vi "WriteCSV.vi"(6 "波形":dbl[][](array[numeric]), 7 "通用数据":string[](array[string]), 9 "任务编号":string, 10 "时间":string, 11 "file path (dialog if empty)":path caption="文件路径 （空时为对话框）") -> ()   [LabVIEW 2018]
uses:
  <vilib>/Utility/file.llb/Write Delimited Spreadsheet (string).vi
  <vilib>/Utility/file.llb/Write Delimited Spreadsheet (DBL).vi
  <vilib>/Utility/file.llb/Read Delimited Spreadsheet (string).vi
panel:
  out "子数组":string[][](array[string])
  out "all rows":string[][](array[string]) caption="所有行"
  # "写入CSV文件\n判断是否需要重新写入还是继续写入"
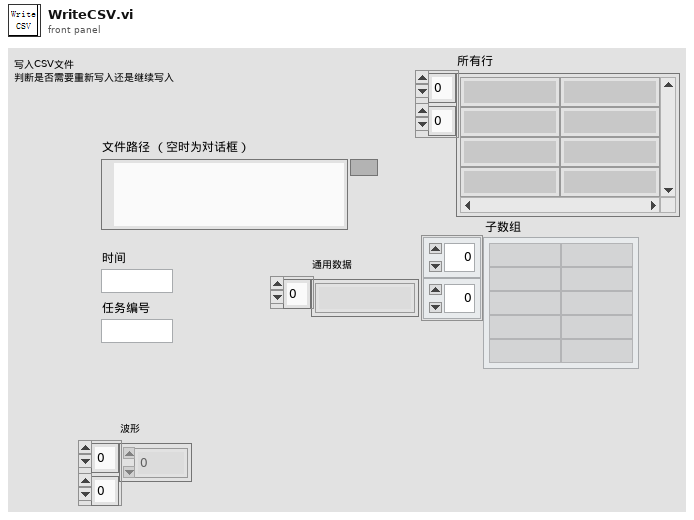
[diagram p1: front panel]
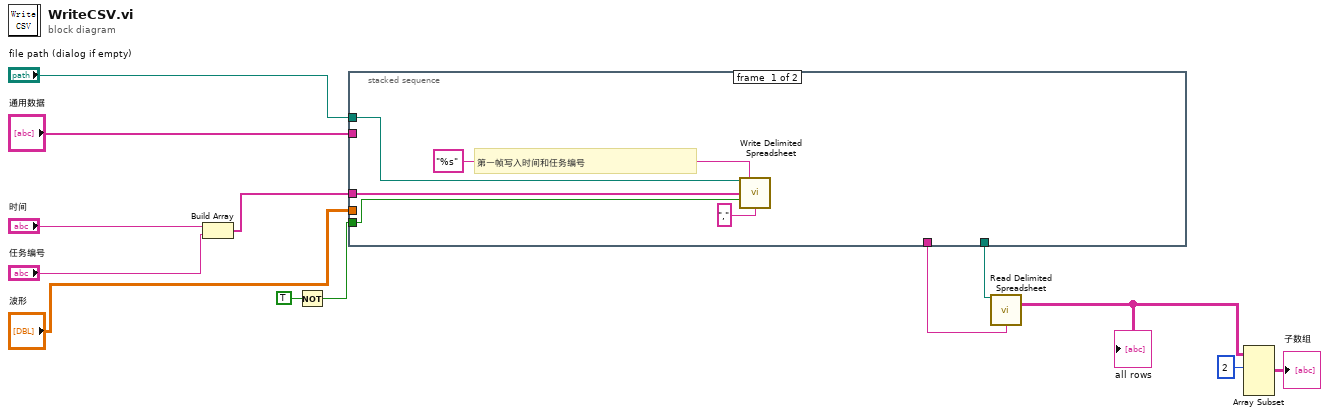
[diagram p0: block diagram]
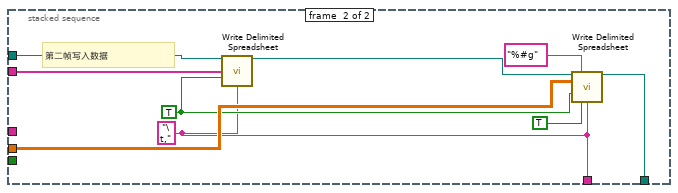
[diagram p2: hidden frame]
diagram:
  n1 = Build Array("时间", "任务编号") -> (w1:string[])
  n2 = Not(x=TRUE ("是否重新写入")) -> (.not. x?=w9:bool)
  n3 = stacked-sequence {
    tunnel: "file path (dialog if empty)" -> [w18 w24]
    tunnel: w9 -> [w16 _]
    tunnel: "波形" -> [_ w27]
    tunnel: "通用数据" -> [_ w25]
    tunnel: [_ w21] -> w6
    tunnel: [_ w19] -> w5
    tunnel: w1 -> [w14 _]
    frame #0 {
      # "第一帧写入时间和任务编号"
      n4 = call-poly <vilib>:"Write Delimited Spreadsheet.vi"("file path (dialog if empty)"=w18, "format (%s)"="%s", "1D data"=w14, "append to file? (new file:F)"=w16, "delimiter (\\t)"="," ("delimiter (\\t)")) -> ()  [unwired: 9 in, 2 out]
    }
    frame #1 {
      w19 = "\t," ("delimiter (\\t)")
      w22 = TRUE ("append to file? (new file:F)")
      # "第二帧写入数据"
      n5 = call-poly <vilib>:"Write Delimited Spreadsheet.vi"("file path (dialog if empty)"=w24, "1D data"=w25, "append to file? (new file:F)"=w22, "delimiter (\\t)"=w19) -> ("new file path (Not A Path if cancelled)"=w23:path)  [unwired: 10 in, 1 out]
      n6 = call-poly <vilib>:"Write Delimited Spreadsheet.vi"("file path (dialog if empty)"=w23, "format (%.3f)"="%#g", "2D data"=w27, "append to file? (new file:F)"=w22, "transpose? (no:F)"=TRUE, "delimiter (\\t)"=w19) -> ("new file path (Not A Path if cancelled)"=w21:path)  [unwired: 8 in, 1 out]
    }
  }
  n7 = call-poly <vilib>:"Read Delimited Spreadsheet.vi"("file path (dialog if empty)"=w6, "delimiter (\\t)"=w5) -> ("all rows"=w4:string[][])  [unwired: 8 in, 5 out]
  "all rows" <- w4
  n8 = Array Subset(array=w4, index (row)=2 ("索引")) -> (→"子数组":string[][])  [unwired: 3 in]
